vi "2L14-n1_limites_de_nc_C_et_A.vi"(2 "S Dem éch de taille n":dbl, 3 "Contrôle (Proba)":dbl, 4 "Alerte (Proba)":dbl, 5 "Valeur Nominale":dbl) -> (0 "Lim. Contrôle":dbl[](array[numeric]), 1 "Lim. Alerte":dbl[](array[numeric]))   [LabVIEW 2010, in "lv_02.lvlib"]
uses:
  lv_02.lvlib
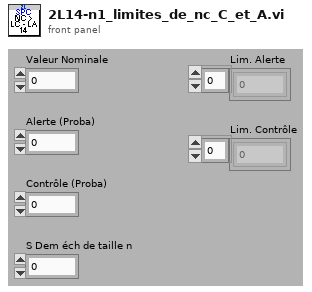
[diagram p1: front panel]
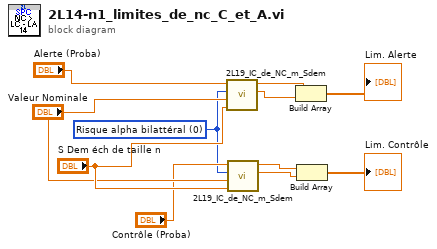
[diagram p0: block diagram]
diagram:
  w1 = u16 0 items=["Risque alpha bilattéral", "Risque alpha à droite", "Risque alpha à gauche"] ("Niveau de confiance")
  n1 = call "2L19_IC_de_NC_m_Sdem.vi"("S dem"="S Dem éch de taille n", "m"="Valeur Nominale", "Niveau de confiance"=w1, "NC"="Alerte (Proba)") -> ("Ic max"=w7:dbl, "Ic min"=w6:dbl)  [unwired: 6 in]
  n2 = call "2L19_IC_de_NC_m_Sdem.vi"("S dem"="S Dem éch de taille n", "m"="Valeur Nominale", "Niveau de confiance"=w1, "NC"="Contrôle (Proba)") -> ("Ic max"=w10:dbl, "Ic min"=w9:dbl)  [unwired: 6 in]
  n3 = Build Array(w6, w7) -> (→"Lim. Alerte":dbl[])
  n4 = Build Array(w9, w10) -> (→"Lim. Contrôle":dbl[])
